vi "Maxigauge on off.vi"() -> ()   [LabVIEW 2020]
panel:
  out "Command success?":string
  out "Sensor 6":bool
  out "Sensor 5":bool
  out "Sensor 4":bool
  out "Sensor 3":bool
  out "Sensor 2":bool
  out "Sensor 1":bool
  in  "bytes":dbl
  in  "Delay":u32=500
  in  "VISA resource name":refnum<visa-resource-name>
  out "error in (no error)":errorcluster
  out "Command sent":string
  in  "Sensor 6":bool
  in  "Sensor 5":bool
  in  "Sensor 4":bool
  in  "Sensor 3":bool
  in  "Sensor 2":bool
  in  "Sensor 1":bool
  # "following Misha's template\nbytes should be set to zero"
  # "End Status"
  # "Request"
  # "If yes, end status indicates the sensor status.\nIf no, end status is all sensors off; command not accepted by Maxigauge"
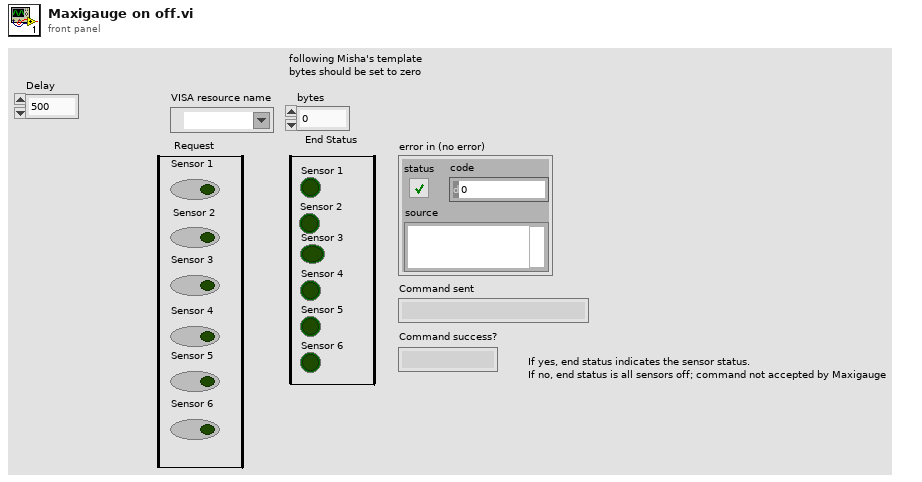
[diagram p1: front panel]
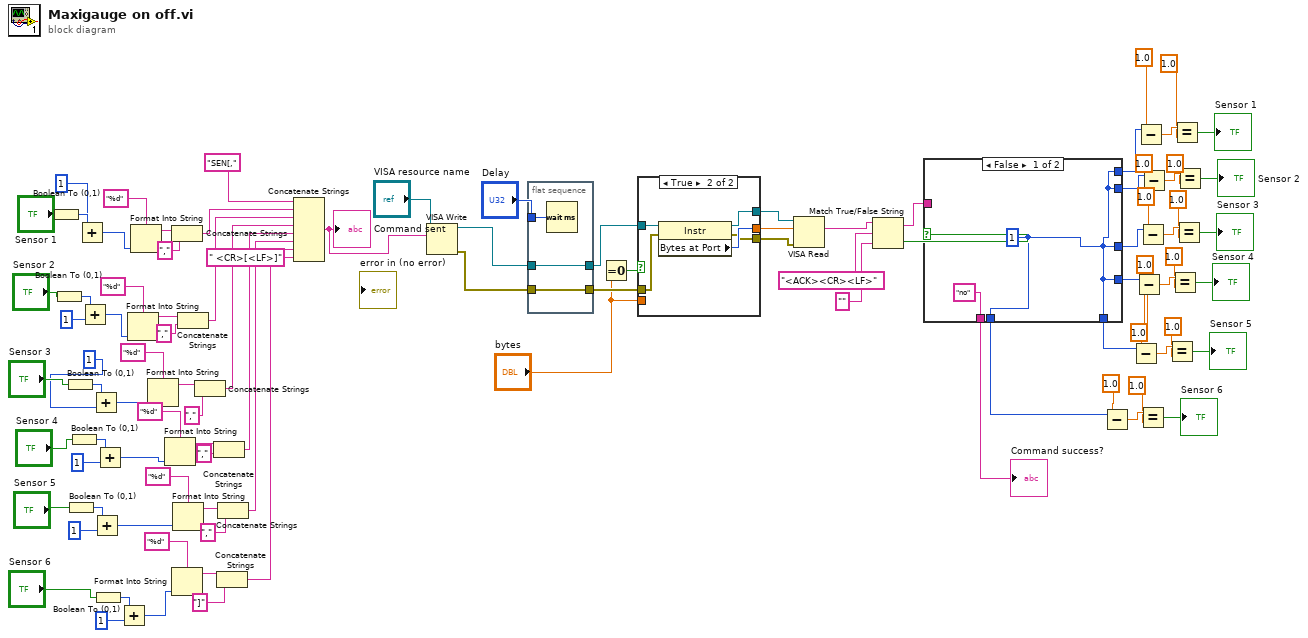
[diagram p0: block diagram]
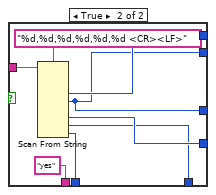
[diagram p2: hidden frame]
diagram:
  n1 = Boolean To (0,1)(Boolean="Sensor 1") -> (0, 1=w66:i16)
  n2 = Boolean To (0,1)(Boolean="Sensor 2") -> (0, 1=w63:i16)
  n3 = Boolean To (0,1)(Boolean="Sensor 3") -> (0, 1=w59:i16)
  n4 = Boolean To (0,1)(Boolean="Sensor 5") -> (0, 1=w51:i16)
  n5 = Boolean To (0,1)(Boolean="Sensor 4") -> (0, 1=w55:i16)
  n6 = Add(x=w66, y=i16 1) -> (x+y=w64:i16)
  n7 = Add(x=w63, y=i16 1) -> (x+y=w60:i16)
  n8 = Add(x=w59, y=i16 1) -> (x+y=w58:i16)
  n9 = Add(x=w51, y=i16 1) -> (x+y=w50:i16)
  n10 = Boolean To (0,1)(Boolean="Sensor 6") -> (0, 1=w47:i16)
  n11 = Add(x=w55, y=i16 1) -> (x+y=w54:i16)
  n12 = Add(x=w47, y=i16 1) -> (x+y=w45:i16)
  n13 = Format Into String(format string="%d", w60) -> (resulting string=w88:string)  [unwired: 2 in, 1 out]
  n14 = Format Into String(format string="%d", w64) -> (resulting string=w91:string)  [unwired: 2 in, 1 out]
  n15 = Format Into String(format string="%d", w58) -> (resulting string=w85:string)  [unwired: 2 in, 1 out]
  n16 = Format Into String(format string="%d", w54) -> (resulting string=w82:string)  [unwired: 2 in, 1 out]
  n17 = Concatenate Strings(w91, "," ("string")) -> (w89:string)
  n18 = Format Into String(format string="%d", w45) -> (resulting string=w76:string)  [unwired: 2 in, 1 out]
  n19 = Format Into String(format string="%d", w50) -> (resulting string=w79:string)  [unwired: 2 in, 1 out]
  n20 = Concatenate Strings(w88, "," ("string")) -> (w84:string)
  n21 = Concatenate Strings(w85, "," ("string")) -> (w83:string)
  n22 = Concatenate Strings(w82, "," ("string")) -> (w80:string)
  n23 = Concatenate Strings(w76, "]" ("string")) -> (w74:string)
  n24 = Concatenate Strings(w79, "," ("string")) -> (w77:string)
  n25 = Concatenate Strings("SEN[," ("string"), w89, w84, w83, w80, w77, w74, " <CR>[<LF>]" ("string")) -> (w72:string)
  "Command sent" <- w72
  n26 = VISA Write(VISA resource name="VISA resource name", write buffer=w72) -> (VISA resource name out=w69:refnum<visa-resource-name>, error out=w70:errorcluster)  [unwired: 1 in, 1 out]
  n27 = flat-sequence {
    tunnel: w70 -> [w100]
    tunnel: [w100] -> w42
    tunnel: w69 -> [w99]
    tunnel: [w99] -> w43
    tunnel: "Delay" -> [w101]
    frame #0 {
      n28 = Wait (ms)(milliseconds to wait=w101) -> ()  [unwired: 1 out]
    }
  }
  n29 = Equal To 0?(x="bytes") -> (x = 0?=w41:bool)
  n30 = case shown="True" w41 {
    tunnel: w43 -> [w104 w109]
    tunnel: w42 -> [w102 w108]
    tunnel: "bytes" -> [w103 _]
    tunnel: [w103 w107] -> w39
    tunnel: [w104 w106] -> w38
    tunnel: [w102 w105] -> w37
    frame False {
    }
    frame True {
      n31 = property class="Instr"(reference=w109, error in=w108) -> (reference out=w106:refnum<visa-resource-name>, error out=w105:errorcluster, "Bytes at Port"=w107:u32)
    }
  }
  n32 = VISA Read(VISA resource name=w38, byte count=w39, error in (no error)=w37) -> (read buffer=w34:string)  [unwired: 3 out]
  n33 = Match True/False String(2:"" ("false string"), 3:"<ACK><CR><LF>" ("true string"), 4:w34) -> (0:w33:bool, 1:w32:string)
  n34 = case shown="False" w33 {
    tunnel: w32 -> [_ w118]
    tunnel: [w111 w117] -> w27
    tunnel: [w111 w116] -> w22
    tunnel: [w111 w116] -> w17
    tunnel: [w111 w115] -> w12
    tunnel: [w111 w114] -> w7
    tunnel: [w111 w113] -> w2
    tunnel: ["no" "yes"] -> w1
    frame False {
      w111 = 1
    }
    frame True {
      n35 = Scan From String(format string="%d,%d,%d,%d,%d,%d <CR><LF>", input string=w118) -> (output 1=w117:i32, output 2=w116:i32, output 4=w115:i32, output 5=w114:i32, output 6=w113:i32)  [unwired: 9 in, 3 out]
    }
  }
  "Command success?" <- w1
  n36 = Subtract(x=w2, y=1.0) -> (x-y=w5:dbl)
  n37 = Subtract(x=w7, y=1.0) -> (x-y=w10:dbl)
  n38 = Subtract(x=w12, y=1.0) -> (x-y=w15:dbl)
  n39 = Subtract(x=w27, y=1.0) -> (x-y=w30:dbl)
  n40 = Subtract(x=w17, y=1.0) -> (x-y=w20:dbl)
  n41 = Equal?(x=w5, y=1.0) -> (x = y?=→"Sensor 6":bool)
  n42 = Subtract(x=w22, y=1.0) -> (x-y=w25:dbl)
  n43 = Equal?(x=w10, y=1.0) -> (x = y?=→"Sensor 5":bool)
  n44 = Equal?(x=w15, y=1.0) -> (x = y?=→"Sensor 4":bool)
  n45 = Equal?(x=w30, y=1.0) -> (x = y?=→"Sensor 1":bool)
  n46 = Equal?(x=w20, y=1.0) -> (x = y?=→"Sensor 3":bool)
  n47 = Equal?(x=w25, y=1.0) -> (x = y?=→"Sensor 2":bool)
